vi "Rohde & Schwarz VNA Set Trigger Mode.vi"(6 "Channel":i8=1 min=1 max=99 step=1, 7 "Rohde & Schwarz VNA":T1, 8 "error in (no error)":errorcluster, 10 "Trigger Mode":T2, 11 "VISA Resource Name":refnum<visa-resource-name>) -> (0 "error out":errorcluster, 3 "dup VISA Resource Name":refnum<visa-resource-name>)   [LabVIEW 2011]
doc: "This VI for the HP8753B Network Analyzers reads the stimulus values. Except when performing log sweeps and freq list sweeps, this VI uses the start and stop values and the number of points to calcuate the stimulus values."
uses:
  TypeDefs/Rohde & Schwarz VNA Trigger Mode.ctl
  TypeDefs/Rohde & Schwarz VNA Instrument Info.ctl
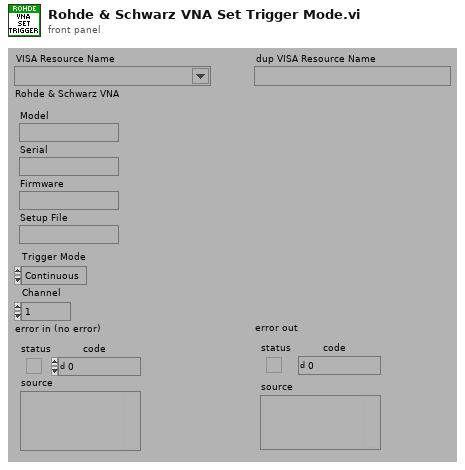
[diagram p1: front panel]
types:
  T1 = typedef "Rohde & Schwarz VNA Instrument Info.ctl" = cluster{"Model":string, "Serial":string, "Firmware":string, "Setup File":string}
  T2 = typedef "Rohde & Schwarz VNA Trigger Mode.ctl" = enum16{"Continuous", "Hold", "Single"}
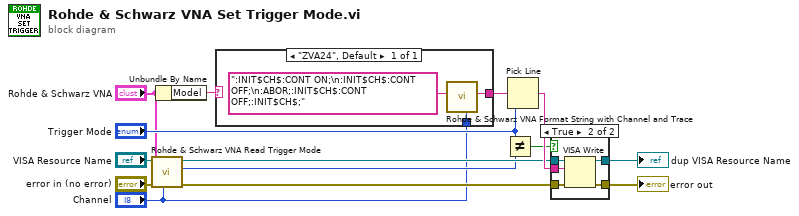
[diagram p0: block diagram]
diagram:
  n1 = call "Rohde & Schwarz VNA Read Trigger Mode.vi"("Channel"="Channel", "Rohde & Schwarz VNA"="Rohde & Schwarz VNA", "error in (no error)"="error in (no error)", "VISA Resource Name"="VISA Resource Name") -> ("error out"=w6:errorcluster, "Trigger Mode"=w4:T2, "dup VISA Resource Name"=w5:refnum<visa-resource-name>)  [unwired: 5 out]
  n2 = Unbundle By Name("Rohde & Schwarz VNA") -> ("Model"=w1:string)
  n3 = case shown="\"ZVA24\", Default" w1 {
    tunnel: [w16] -> w8
    tunnel: "Channel" -> [w15]
    frame "ZVA24", Default {
      n4 = call "Rohde & Schwarz VNA Format String with Channel and Trace.vi"("Trace"=w15, "String"=":INIT$CH$:CONT ON;\n:INIT$CH$:CONT OFF;\n:ABOR;:INIT$CH$:CONT OFF;:INIT$CH$;") -> ("String Out"=w16:string)  [unwired: 1 in, 6 out]
    }
  }
  n5 = Not Equal?(x="Trigger Mode", y=w4) -> (x != y?=w7:bool)
  n6 = Pick Line(multi-line string=w8, line index="Trigger Mode") -> (output string=w9:string)  [unwired: 1 out]
  n7 = case shown="True" w7 {
    tunnel: w6 -> [w18 w24]
    tunnel: w5 -> [w19 w23]
    tunnel: w9 -> [_ w22]
    tunnel: [w19 w21] -> w14
    tunnel: [w18 w20] -> w13
    frame False {
    }
    frame True {
      n8 = VISA Write(VISA resource name=w23, write buffer=w22, error in (no error)=w24) -> (VISA resource name out=w21:refnum<visa-resource-name>, error out=w20:errorcluster)  [unwired: 1 out]
    }
  }
  "dup VISA Resource Name" <- w14
  "error out" <- w13
